vi "Timev2.vi"(1 "Timing Data":i32[](array[numeric]), 8 "error in (no error)":errorcluster, 10 "Control In":T1, 11 "CAD Dispense in":refnum<class "CAD Dispense.lvclass">) -> (0 "error out":errorcluster, 2 "Control Out":T1, 3 "CAD Dispense Out":refnum<class "CAD Dispense.lvclass">)   [LabVIEW 2020, in "CAD Dispense.lvclass"]
uses:
  CAD Dispense.lvclass
  Aerotech.lvlib
  Program Files (x86)/Aerotech/A3200/LabVIEW/2010/Motion/MoveIncSingle.vi
  Controller/Motion/Motion.lvclass
  Controller/I-O/I-O.lvclass
  Controller/Dispenser/Dispenser.lvclass
  C:/Program Files (x86)/Aerotech/A3200/LabVIEW/2010/Bin/Aerotech.A3200.dll
  Program Files (x86)/Aerotech/A3200/LabVIEW/2010/Bin/Aerotech.A3200.dll
  Controller/Controllers.ctl
  Controller/Controller.lvclass
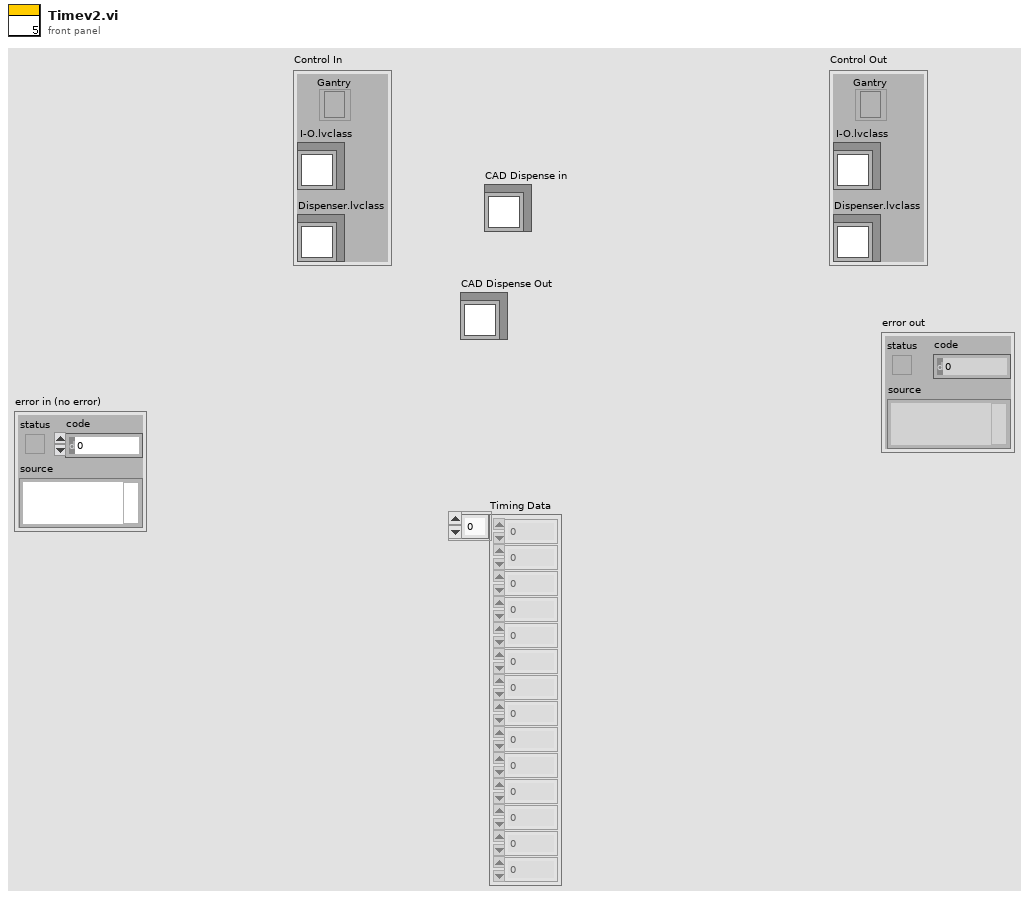
[diagram p1: front panel]
types:
  T1 = typedef "Controller.lvclass/Controllers.ctl" = cluster{"I-O.lvclass":refnum<class "I-O.lvclass">, "Dispenser.lvclass":refnum<class "Dispenser.lvclass">, "Gantry":refnum<k24>}
  T2 = cluster{"Motion":dbl[][], "Center":dbl[], "CW/CCW":dbl, "Dispense Type":enum16{"N-gon", "Square", "Arc", "Dot", "Line", "Circle"}}[]
  T3 = cluster{"Motion":dbl[][], "Center":dbl[], "CW/CCW":dbl, "Dispense Type":enum16{"N-gon", "Square", "Arc", "Dot", "Line", "Circle"}}
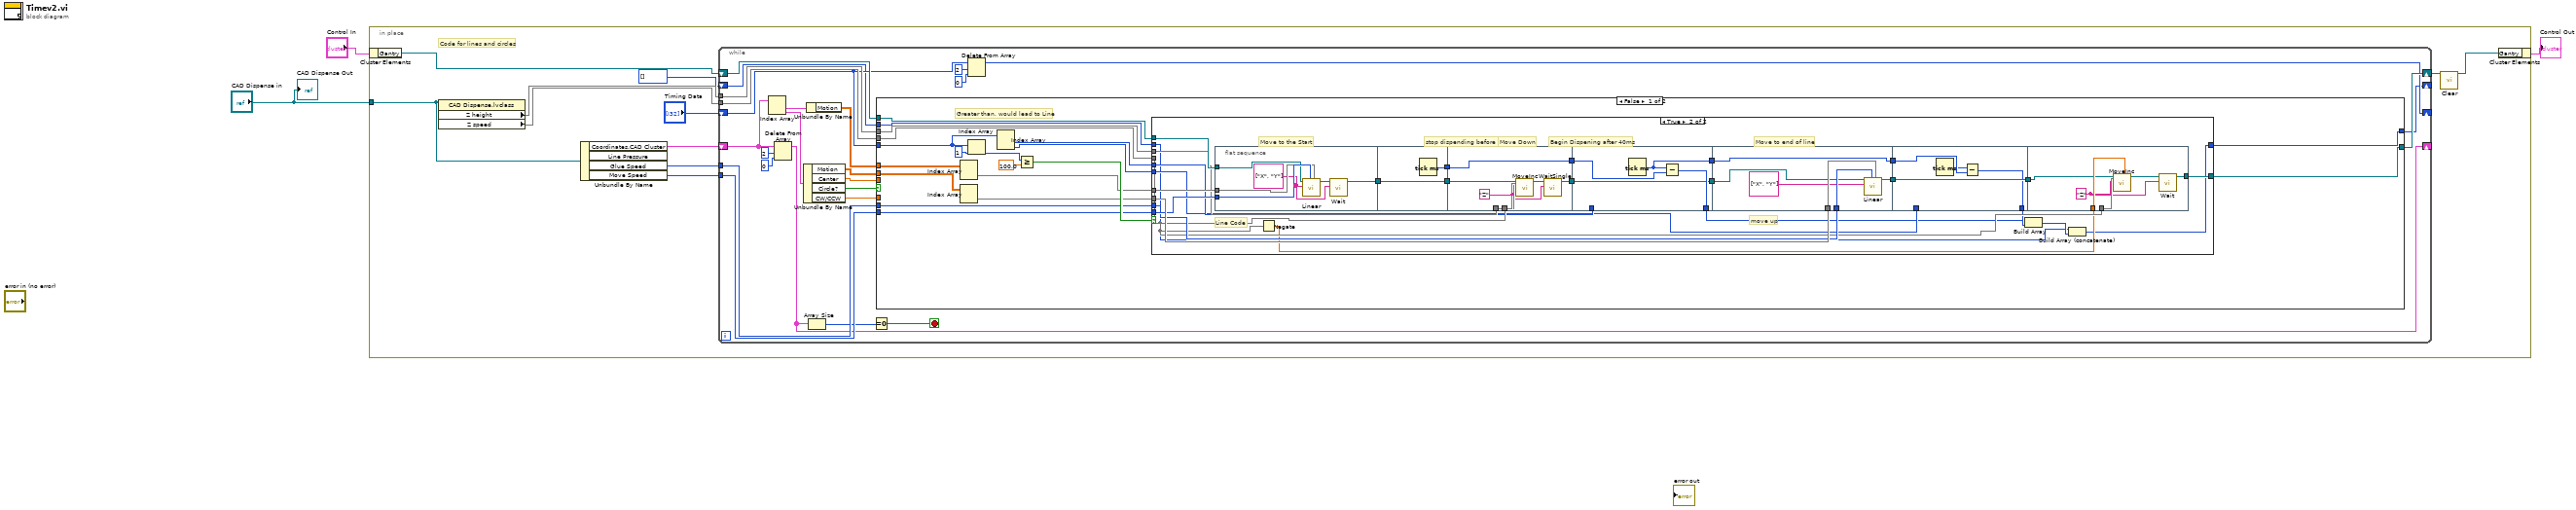
[diagram p0: block diagram]
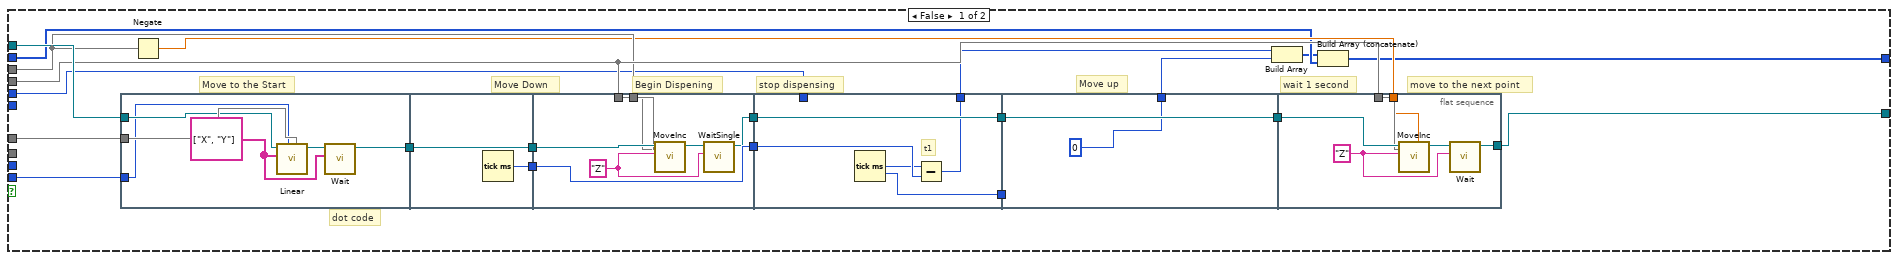
[diagram p2: hidden frame]
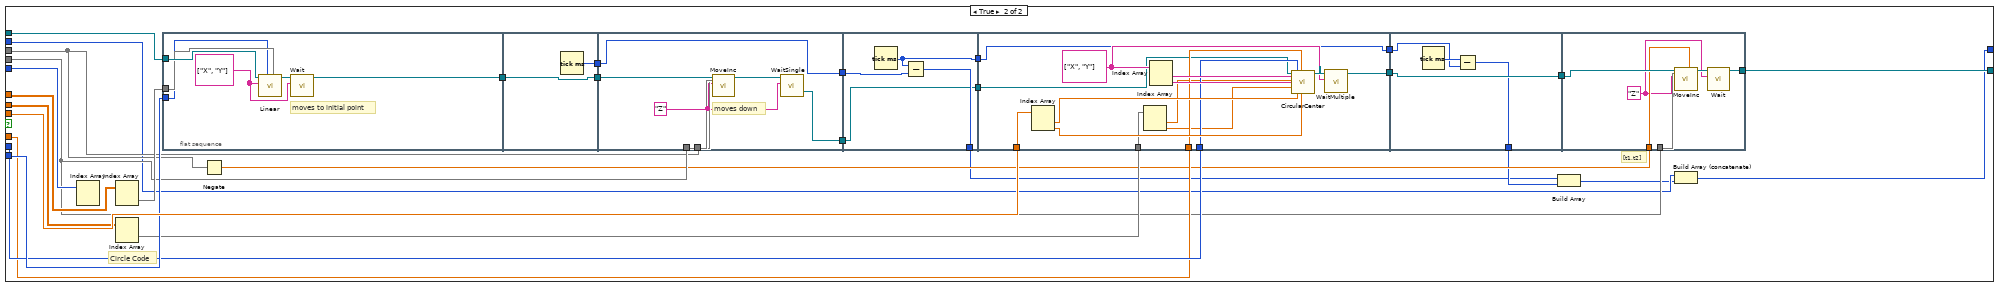
[diagram p3: hidden frame]
diagram:
  n1 = in-place {
    in-place-border: "CAD Dispense in" -> [w5]
    # "Code for lines and circles"
    n2 = in-place-cluster #1("Control In") -> ("Gantry"=w7:refnum<k24>)
    n3 = property class="CAD Dispense.lvclass"(reference=w5) -> ("Z height"=w10, "Z speed"=w11)  [unwired: 1 in, 2 out]
    n4 = Unbundle By Name "Unbundle By Name"(w5) -> ("Coordinates.CAD Cluster"=w12:T2, "Glue Speed"=w9:i32, "Move Speed"=w14:i32)  [unwired: 1 out]
    n5 = while {
      tunnel: w14 -> [w36]
      shift-right: [w33] -> w8
      shift-left: w7 -> [w37]
      shift-right: [w23] -> _
      shift-left: "Timing Data" -> [w24]
      shift-right: [w19] -> _
      shift-left: w12 -> [w20]
      tunnel: w11 -> [w32]
      tunnel: w10 -> [w31]
      tunnel: w9 -> [w30]
      shift-right: [w15] -> _
      shift-left: i32[] [] -> [w16]
      stop <- w17 stop-if-true
      n6 = Index Array(array=w20) -> (element #1=w39:T3, element #2=w35:T3)  [unwired: 2 in]
      n7 = Delete From Array(array=w20, length=2, index=0) -> (array with subset deleted=w19:T2)  [unwired: 1 out]
      n8 = Unbundle By Name(w35) -> ("Motion"=w34:dbl[][], "Center"=w28:dbl[], "Circle?"=w29:bool, "CW/CCW"=w27:dbl)
      n9 = Unbundle By Name(w39) -> ("Motion"=w38:dbl[][])
      n10 = Array Size(array=w19) -> (size(s)=w18:i32)
      n11 = Equal To 0?(x=w18) -> (x = 0?=w17:bool)
      n12 = case shown="False" w29 {
        tunnel: w24 -> [w44 w191]
        tunnel: w28 -> [_ w196]
        tunnel: w38 -> [w54 w195]
        tunnel: w37 -> [w50 w194]
        tunnel: w36 -> [w48 w193]
        tunnel: w34 -> [w51 w187]
        tunnel: [w49 w192] -> w33
        tunnel: w32 -> [w46 w185]
        tunnel: w31 -> [w47 w184]
        tunnel: w30 -> [w45 w189]
        tunnel: w27 -> [_ w188]
        tunnel: w16 -> [w41 w173]
        tunnel: [w40 w171] -> w15
        frame False {
          # "Greater than, would lead to Line"
          n13 = Index Array(array=w54) -> (element=w53:dbl[])  [unwired: 2 in]
          n14 = Index Array(array=w51) -> (element=w52:dbl[])  [unwired: 2 in]
          n15 = Index Array(array=w44, index=1) -> (element=w57:i32)
          n16 = Index Array(array=w44) -> (element #1=w43:i32, element #2=w42:i32)  [unwired: 2 in]
          n17 = Greater Or Equal?(x=w57, y=100.0) -> (x >= y?=w55:bool)
          n18 = case shown="True" w55 {
            tunnel: w53 -> [w70 w132]
            tunnel: w52 -> [_ w131]
            tunnel: w50 -> [w79 w130]
            tunnel: [w75 w128] -> w49
            tunnel: w48 -> [w74 w127]
            tunnel: w47 -> [w72 w125]
            tunnel: w46 -> [w73 w124]
            tunnel: w45 -> [_ w126]
            tunnel: w43 -> [w69 w122]
            tunnel: w42 -> [_ w121]
            tunnel: w41 -> [w62 w112]
            tunnel: [w60 w111] -> w40
            frame False {
              # "dot code"
              # "stop dispensing"
              # "move to the next point"
              # "wait 1 second"
              # "Move up"
              # "Begin Dispening"
              # "Move Down"
              # "Move to the Start"
              n19 = flat-sequence {
                tunnel: w79 -> [w83]
                tunnel: [w85] -> w68
                tunnel: w74 -> [w81]
                tunnel: w70 -> [w84]
                tunnel: w68 -> [w87]
                tunnel: [w87] -> w67
                tunnel: [w86] -> w65
                tunnel: w67 -> [w94]
                tunnel: [w89] -> w78
                tunnel: w72 -> [w93]
                tunnel: w73 -> [w92]
                tunnel: [w91] -> w66
                tunnel: w65 -> [w91]
                tunnel: w78 -> [w98]
                tunnel: [w98] -> w77
                tunnel: w69 -> [_]
                tunnel: w66 -> [w97]
                tunnel: [w96] -> w64
                tunnel: [w95] -> w59
                tunnel: [w100] -> w76
                tunnel: [0] -> w63
                tunnel: w77 -> [w100]
                tunnel: w64 -> [_]
                tunnel: [w106] -> w75
                tunnel: w71 -> [w102]
                tunnel: w73 -> [w103]
                tunnel: w76 -> [w104]
                frame #0 {
                  w80 = string[] ["X", "Y"] ("axis names")
                  n20 = call "Linear.vi"("distances"=w84, "speed"=w81, "axis names"=w80, "controller in"=w83) -> ("controller out"=w82:refnum<k24>)  [unwired: 6 in, 1 out]
                  n21 = call-poly "Wait.vi"("axis names"=w80, "controller in"=w82) -> ("controller out"=w85:refnum<k24>)  [unwired: 7 in, 2 out]
                }
                frame #1 {
                  n22 = Tick Count (ms)() -> (millisecond timer value=w86:u32)
                }
                frame #2 {
                  w88 = "Z" ("axis name")
                  n23 = call-poly "MoveInc.vi"("distance"=w93, "speed"=w92, "axis name"=w88, "controller in"=w94) -> ("controller out"=w90:refnum<k24>)  [unwired: 6 in, 1 out]
                  n24 = call "WaitSingle.vi"("axis name"=w88, "controller in"=w90) -> ("controller out"=w89:refnum<k24>)  [unwired: 7 in, 2 out]
                }
                frame #3 {
                  # "t1"
                  n25 = Tick Count (ms)() -> (millisecond timer value=w96:u32)
                  n26 = Subtract(x=w96, y=w97) -> (x-y=w95:u32)
                }
                frame #4 {
                }
                frame #5 {
                  w101 = "Z" ("axis name")
                  n27 = call-poly "MoveInc.vi"("distance"=w102, "speed"=w103, "axis name"=w101, "controller in"=w104) -> ("controller out"=w105:refnum<k24>)  [unwired: 6 in, 1 out]
                  n28 = call-poly "Wait.vi"("axis name"=w101, "controller in"=w105) -> ("controller out"=w106:refnum<k24>)  [unwired: 7 in, 2 out]
                }
              }
              n29 = Negate(x=w72) -> (-x=w71:dbl)
              n30 = Build Array(w59, w63) -> (w61:u32[])
              n31 = Build Array (concatenate)(w61, w62) -> (w60:u32[])
            }
            frame True {
              # "Move to end of line"
              # "move up"
              # "stop dispending before 40ms"
              # "Begin Dispening after 40ms"
              # "Move Down"
              # "Move to the Start"
              # "Line Code"
              n32 = flat-sequence {
                tunnel: w132 -> [w136]
                tunnel: w130 -> [w133]
                tunnel: [w138] -> w120
                tunnel: w127 -> [w137]
                tunnel: w120 -> [w140]
                tunnel: [w140] -> w119
                tunnel: [w139] -> w118
                tunnel: w119 -> [w147]
                tunnel: w125 -> [w146]
                tunnel: w124 -> [w145]
                tunnel: w118 -> [w144]
                tunnel: [w144] -> w117
                tunnel: [w141] -> w110
                tunnel: w117 -> [w151]
                tunnel: w122 -> [_]
                tunnel: [w150] -> w115
                tunnel: [w149] -> w107
                tunnel: w110 -> [w148]
                tunnel: [w148] -> w109
                tunnel: w131 -> [w156]
                tunnel: [w157] -> w129
                tunnel: w126 -> [w155]
                tunnel: [w153] -> w116
                tunnel: w115 -> [w153]
                tunnel: w109 -> [w152]
                tunnel: w129 -> [w159]
                tunnel: w121 -> [_]
                tunnel: w116 -> [w161]
                tunnel: [w158] -> w114
                tunnel: [w159] -> w108
                tunnel: [w167] -> w128
                tunnel: w123 -> [w164]
                tunnel: w124 -> [w165]
                tunnel: w108 -> [w162]
                frame #0 {
                  w134 = string[] ["X", "Y"] ("axis names")
                  n33 = call "Linear.vi"("distances"=w136, "speed"=w137, "axis names"=w134, "controller in"=w133) -> ("controller out"=w135:refnum<k24>)  [unwired: 6 in, 1 out]
                  n34 = call-poly "Wait.vi"("axis names"=w134, "controller in"=w135) -> ("controller out"=w138:refnum<k24>)  [unwired: 7 in, 2 out]
                }
                frame #1 {
                  n35 = Tick Count (ms)() -> (millisecond timer value=w139:u32)
                }
                frame #2 {
                  w142 = "Z" ("axis name")
                  n36 = call-poly "MoveInc.vi"("distance"=w146, "speed"=w145, "axis name"=w142, "controller in"=w147) -> ("controller out"=w143:refnum<k24>)  [unwired: 6 in, 1 out]
                  n37 = call "WaitSingle.vi"("axis name"=w142, "controller in"=w143) -> ("controller out"=w141:refnum<k24>)  [unwired: 7 in, 2 out]
                }
                frame #3 {
                  n38 = Tick Count (ms)() -> (millisecond timer value=w150:u32)
                  n39 = Subtract(x=w150, y=w151) -> (x-y=w149:u32)
                }
                frame #4 {
                  n40 = call "Linear.vi"("distances"=w156, "speed"=w155, "axis names"=string[] ["X", "Y"], "controller in"=w152) -> ("controller out"=w157:refnum<k24>)  [unwired: 6 in, 1 out]
                }
                frame #5 {
                  n41 = Tick Count (ms)() -> (millisecond timer value=w160:u32)
                  n42 = Subtract(x=w160, y=w161) -> (x-y=w158:u32)
                }
                frame #6 {
                  w163 = "Z" ("axis name")
                  n43 = call-poly "MoveInc.vi"("distance"=w164, "speed"=w165, "axis name"=w163, "controller in"=w162) -> ("controller out"=w166:refnum<k24>)  [unwired: 6 in, 1 out]
                  n44 = call-poly "Wait.vi"("axis name"=w163, "controller in"=w166) -> ("controller out"=w167:refnum<k24>)  [unwired: 7 in, 2 out]
                }
              }
              n45 = Negate(x=w124) -> (-x=w123:dbl)
              n46 = Build Array(w107, w114) -> (w113:u32[])
              n47 = Build Array (concatenate) "Build Array"(w112, w113) -> (w111:u32[])
            }
          }
        }
        frame True {
          # "[t1,t2]"
          # "Circle Code"
          n48 = Index Array(array=w191) -> ()  [unwired: 2 in, 2 out]
          n49 = Index Array(array=w195) -> (element=w190:dbl[])  [unwired: 2 in]
          n50 = Index Array(array=w187) -> (element=w186:dbl[])  [unwired: 2 in]
          n51 = flat-sequence {
            tunnel: w194 -> [w201]
            tunnel: w193 -> [w197]
            tunnel: [w202] -> w182
            tunnel: w190 -> [w198]
            tunnel: w182 -> [w204]
            tunnel: [w204] -> w181
            tunnel: [w203] -> w179
            tunnel: w181 -> [w211]
            tunnel: [w207] -> w180
            tunnel: w185 -> [w210]
            tunnel: w184 -> [w209]
            tunnel: w179 -> [w205]
            tunnel: [w205] -> w178
            tunnel: w180 -> [w212]
            tunnel: w178 -> [w215]
            tunnel: [w214] -> w175
            tunnel: [w213] -> w168
            tunnel: [w212] -> w170
            tunnel: w196 -> [w228]
            tunnel: [w218] -> w177
            tunnel: w189 -> [w225]
            tunnel: w188 -> [w224]
            tunnel: w186 -> [w223]
            tunnel: [w217] -> w176
            tunnel: w175 -> [w217]
            tunnel: w170 -> [w216]
            tunnel: w177 -> [w234]
            tunnel: [w234] -> w174
            tunnel: w176 -> [w232]
            tunnel: [w231] -> w169
            tunnel: w174 -> [w240]
            tunnel: [w238] -> w192
            tunnel: w185 -> [w237]
            tunnel: w183 -> [w236]
            frame #0 {
              w199 = string[] ["X", "Y"] ("axis names")
              # "moves to initial point"
              n52 = call "Linear.vi"("distances"=w198, "speed"=w197, "axis names"=w199, "controller in"=w201) -> ("controller out"=w200:refnum<k24>)  [unwired: 6 in, 1 out]
              n53 = call-poly "Wait.vi"("axis names"=w199, "controller in"=w200) -> ("controller out"=w202:refnum<k24>)  [unwired: 7 in, 2 out]
            }
            frame #1 {
              n54 = Tick Count (ms)() -> (millisecond timer value=w203:u32)
            }
            frame #2 {
              w206 = "Z" ("axis name")
              # "moves down"
              n55 = call-poly "MoveInc.vi"("distance"=w210, "speed"=w209, "axis name"=w206, "controller in"=w211) -> ("controller out"=w208:refnum<k24>)  [unwired: 6 in, 1 out]
              n56 = call "WaitSingle.vi"("axis name"=w206, "controller in"=w208) -> ("controller out"=w207:refnum<k24>)  [unwired: 7 in, 2 out]
            }
            frame #3 {
              n57 = Tick Count (ms)() -> (millisecond timer value=w214:u32)
              n58 = Subtract(x=w214, y=w215) -> (x-y=w213:u32)
            }
            frame #4 {
              w219 = string[] ["X", "Y"] ("array")
              n59 = Index Array "Index Array"(array=w228) -> (element #1=w227:dbl, element #2=w226:dbl)  [unwired: 2 in]
              n60 = Index Array(array=w223) -> (element #1=w222:dbl, element #2=w221:dbl)  [unwired: 2 in]
              n61 = Index Array(array=w219) -> (element #1=w230:string, element #2=w229:string)  [unwired: 2 in]
              n62 = call "CircularCenter.vi"("controller in"=w216, "axis 1 name"=w230, "axis 1 endpoint"=w222, "axis 2 name"=w229, "axis 2 endpoint"=w221, "speed"=w225, "axis 1 center point"=w227, "direction"=w224, "axis 2 center point"=w226) -> ("controller out"=w220:refnum<k24>)  [unwired: 9 in, 1 out]
              n63 = call "WaitMultiple.vi"("axis names"=w219, "controller in"=w220) -> ("controller out"=w218:refnum<k24>)  [unwired: 7 in, 2 out]
            }
            frame #5 {
              n64 = Tick Count (ms)() -> (millisecond timer value=w233:u32)
              n65 = Subtract(x=w233, y=w232) -> (x-y=w231:u32)
            }
            frame #6 {
              w235 = "Z" ("axis name")
              n66 = call-poly "MoveInc.vi"("distance"=w236, "speed"=w237, "axis name"=w235, "controller in"=w240) -> ("controller out"=w239:refnum<k24>)  [unwired: 6 in, 1 out]
              n67 = call-poly "Wait.vi"("axis name"=w235, "controller in"=w239) -> ("controller out"=w238:refnum<k24>)  [unwired: 7 in, 2 out]
            }
          }
          n68 = Negate(x=w184) -> (-x=w183:dbl)
          n69 = Build Array "Build Array"(w168, w169) -> (w172:u32[])
          n70 = Build Array (concatenate) "Build Array"(w173, w172) -> (w171:u32[])
        }
      }
      n71 = Delete From Array(array=w24, length=2, index=0) -> (array with subset deleted=w23:i32[])  [unwired: 1 out]
    }
    n72 = call "Clear.vi"("Gantry 2"=w8) -> ("Gantry 3"=w6:refnum<k24>)  [unwired: 9 in, 1 out]
    n73 = in-place-cluster #1("Gantry"=w6) -> (→"Control Out":T1)
  }
  "CAD Dispense Out" <- "CAD Dispense in"
